vi "PID (DBL Array).vi"(6 "reinitialize? (F)":bool, 7 "output range":cluster{"output high":dbl, "output low":dbl}[](array[cluster])=[{"output high"=100.0, "output low"=-100.0}] {"output low" format="%.2f"; "output high" format="%.2f"}, 8 "dt (s)":dbl=-1.0 format="%.3f", 9 "PID gains":T1(array[cluster])=[{"proportional gain (Kc)"=1.0, "integral time (Ti, min)"=0.01, "derivative time (Td, min)"=0.0}] {"derivative time (Td, min)" format="%.3f"; "integral time (Ti, min)" format="%.3f"; "proportional gain (Kc)" format="%.3f"}, 10 "process variable":dbl[](array[numeric])=[0.0] format="%.2f", 11 "setpoint":dbl[](array[numeric])=[0.0] format="%.2f") -> (0 "dt out (s)":dbl format="%.3f", 3 "output":dbl[](array[numeric]) format="%.2f")   [LabVIEW 2020, in "NI_PID_pid.lvlib"]
doc: "Implements a PID controller using a PID algorithm for simple PID applications or high speed control applications that require an efficient algorithm. The PID algorithm features control output range limiting with integrator anti-windup and bumpless controller output for PID gain changes. Use the DBL instance of this VI to implement a single control loop. Use the DBL Array instance to implement parallel multi-loop control."
uses:
  <vilib>/addons/control/pid/NI_PID_pid.lvlib
  <vilib>/addons/control/pid/lvpidtkt.dll
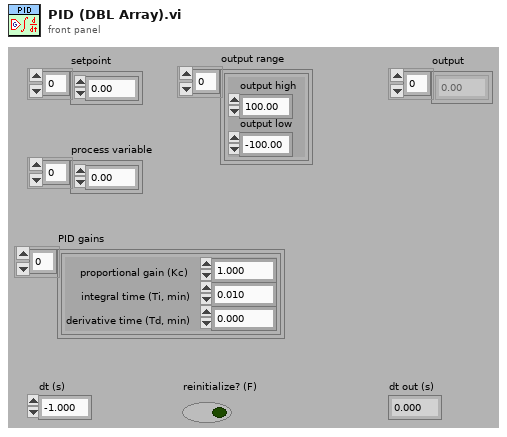
[diagram p1: front panel]
types:
  T1 = cluster{"proportional gain (Kc)":dbl, "integral time (Ti, min)":dbl, "derivative time (Td, min)":dbl}[]
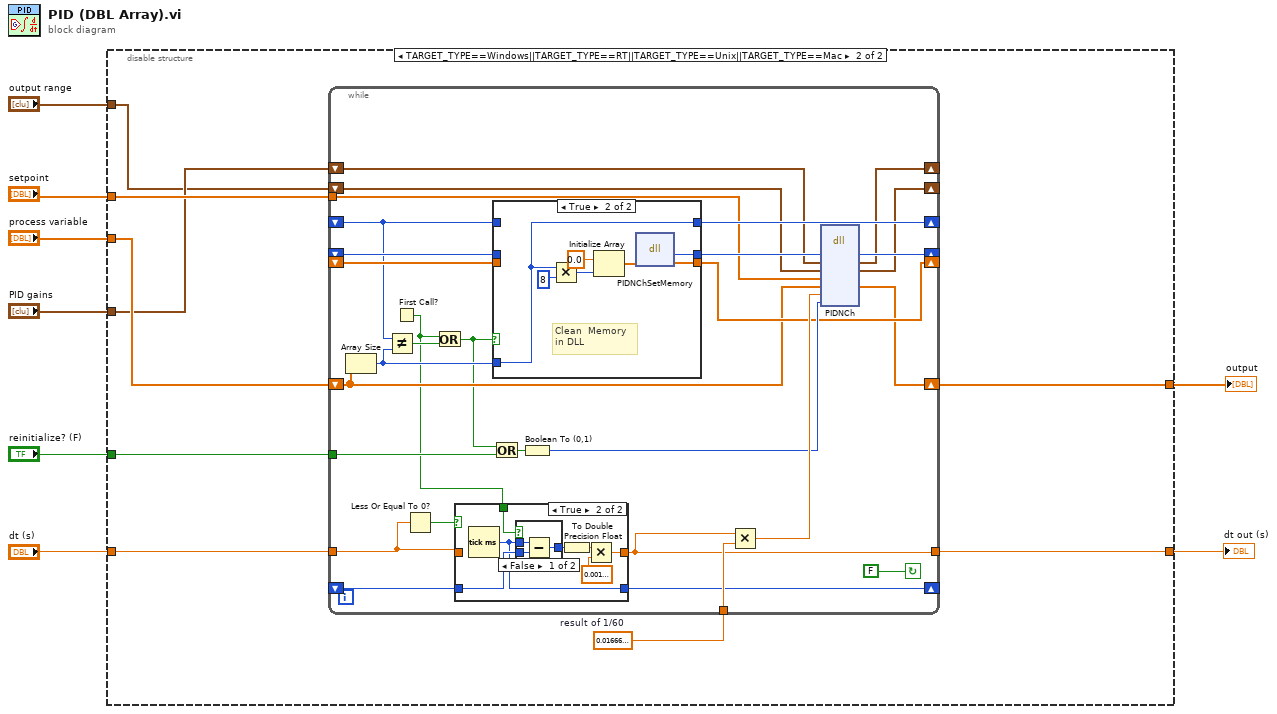
[diagram p0: block diagram]
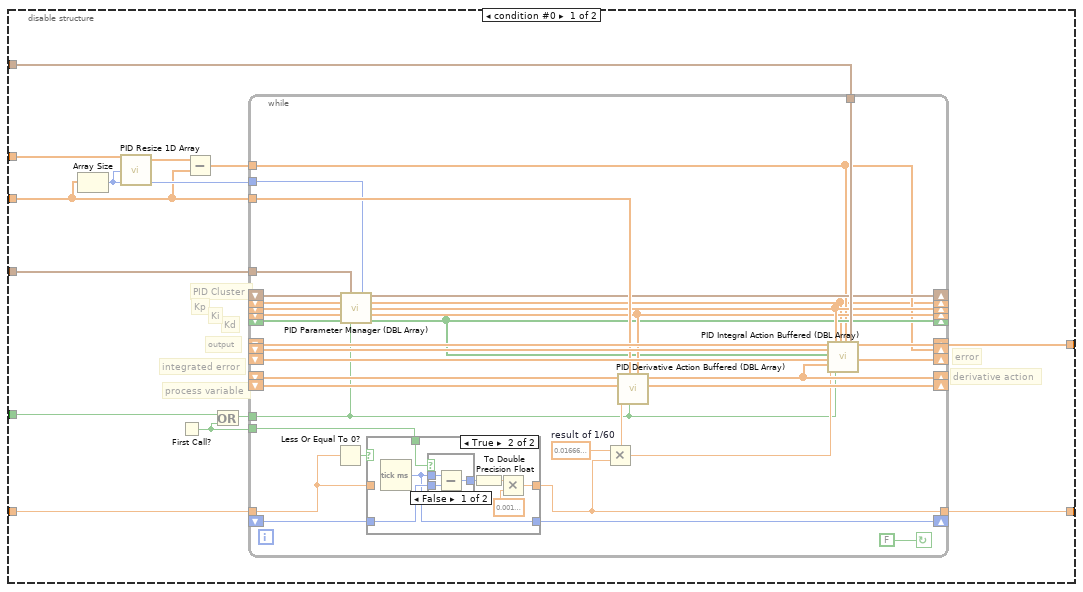
[diagram p2: hidden frame]
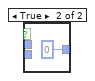
[diagram p4: hidden frame]
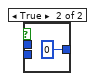
[diagram p6: hidden frame]
diagram:
  n1 = disable-structure shown="TARGET_TYPE==Windows||TARGET_TYPE==RT||TARGET_TYPE==Unix||TARGET_TYPE==Mac" {
    disable-tunnel: "reinitialize? (F)" -> [w21 w72]
    disable-tunnel: [w20 w75] -> w7
    disable-tunnel: [w19 w76] -> w6
    disable-tunnel: "dt (s)" -> [w18 w77]
    disable-tunnel: "output range" -> [w15 w69]
    disable-tunnel: "setpoint" -> [w13 w74]
    disable-tunnel: "process variable" -> [w10 w73]
    disable-tunnel: "PID gains" -> [w14 w70]
    frame condition #0 {
      # "Kd"
      # "Ki"
      # "Kp"
      # "PID Cluster"
      # "integrated error"
      # "error"
      # "output"
      # "process variable"
      # "derivative action"
      n2 = Array Size(array=w10) -> (size(s)=w12:i32)
      n3 = call <vilib>:"PID Resize 1D Array.vi"("array size"=w12, "input array"=w13) -> ("output array"=w11:dbl[])  [unwired: 3 in]
      n4 = First Call?() -> (First Call?: T/F=w16:bool)
      n5 = Subtract(x=w11, y=w10) -> (x-y=w9:dbl[])
      n6 = Or(x=w21, y=w16) -> (x .or. y?=w17:bool)
      n7 = while {
        tunnel: w17 -> [w25]
        shift-left: _ -> [w42]
        shift-right: [w41] -> _
        shift-right: [w46] -> _
        shift-left: _ -> [w47]
        shift-right: [w54] -> _
        shift-left: _ -> [w48]
        shift-right: [w53] -> w20
        shift-left: _ -> [w51]
        shift-right: [w23] -> _
        shift-left: _ -> [w52]
        shift-right: [w50] -> _
        shift-left: _ -> [w49]
        tunnel: w18 -> [w38]
        tunnel: [w40] -> w19
        tunnel: w10 -> [w36]
        tunnel: w12 -> [w24]
        tunnel: w15 -> [w43]
        tunnel: w16 -> [w37]
        shift-right: [w26] -> _
        shift-left: _ -> [w35]
        shift-right: [w27] -> _
        shift-left: _ -> [w34]
        shift-right: [w28] -> _
        shift-left: _ -> [w33]
        shift-right: [w22] -> _
        shift-left: _ -> [w32]
        shift-right: [w31] -> _
        shift-left: _ -> [w30]
        tunnel: w14 -> [w29]
        tunnel: w9 -> [w23]
        stop <- FALSE continue-if-true
        w44 = 0.016666666666666666  # result of 1/60
        n8 = Less Or Equal To 0?(x=w38) -> (x <= 0?=w39:bool)
        n9 = call <vilib>:"PID Parameter Manager (DBL Array).vi"("previous PID gains"=w30, "PID gains"=w29, "process variable size"=w24, "previous Kp"=w32, "previous Ki"=w33, "previous Kd"=w34, "previous PID Gains equal ?"=w35, "initialize"=w25) -> ("PID Parameter Out"=w31:T1, "Kp"=w22:dbl[], "Ki"=w28:dbl[], "Kd"=w27:dbl[], "PID Gains equal ?"=w26:bool[])  [unwired: 2 in, 1 out]
        n10 = case shown="True" w39 {
          tunnel: [w57 w61] -> w40
          tunnel: w42 -> [w56 w60]
          tunnel: [w56 w59] -> w41
          tunnel: w38 -> [w57 _]
          tunnel: w37 -> [_ w58]
          frame False {
          }
          frame True {
            n11 = Tick Count (ms)() -> (millisecond timer value=w59:u32)
            n12 = case shown="False" w58 {
              tunnel: [w67 u32 0] -> w63
              tunnel: w60 -> [w66 _]
              tunnel: w59 -> [w65 _]
              frame False {
                n13 = Subtract(x=w65, y=w66) -> (x-y=w67:u32)
              }
              frame True {
              }
            }
            n14 = To Double Precision Float(number=w63) -> (double precision float=w62:dbl)
            n15 = Multiply(x=w62, y=0.0010000000474974513) -> (x*y=w61:dbl)
          }
        }
        n16 = Multiply(x=w44, y=w40) -> (x*y=w45:dbl)
        n17 = call <vilib>:"PID Derivative Action Buffered (DBL Array).vi"("Kd"=w27, "initialize (F)"=w25, "process variable"=w36, "dt (min)"=w45, "previous  process variable"=w48, "previous derivative action"=w47) -> ("process variable buffer"=w54:dbl[], "derivative action"=w46:dbl[])  [unwired: 4 in]
        n18 = call <vilib>:"PID Integral Action Buffered (DBL Array).vi"("previous output"=w51, "previous error"=w52, "PID Gains equal?"=w26, "previous integrated error"=w49, "previous derivative action"=w46, "dt (min)"=w45, "Ki"=w28, "initialize (F)"=w25, "proportional action"=w22, "error"=w23, "output range"=w43) -> ("output"=w53:dbl[], "integrated error out"=w50:dbl[])  [unwired: 7 in]
      }
    }
    frame condition #1 (active) {
      w71 = 0.016666666666666666  # result of 1/60
      n19 = while {
        shift-right: [w81] -> _
        shift-left: _ -> [w82]
        shift-right: [w101] -> _
        shift-left: _ -> [w102]
        shift-right: [w99] -> _
        shift-left: _ -> [w98]
        shift-right: [w97] -> _
        shift-left: _ -> [w95]
        shift-right: [w91] -> _
        shift-left: w70 -> [w93]
        shift-right: [w90] -> _
        shift-left: w69 -> [w92]
        shift-right: [w88] -> w75
        shift-left: w73 -> [w89]
        tunnel: w77 -> [w80]
        tunnel: w74 -> [w86]
        tunnel: [w78] -> w76
        tunnel: w72 -> [w85]
        tunnel: w71 -> [w84]
        stop <- FALSE continue-if-true
        n20 = Array Size(array=w89) -> (size(s)=w96:i32)
        n21 = Not Equal?(x=w95, y=w96) -> (x != y?=w94:bool)
        n22 = First Call?() -> (First Call?: T/F=w79:bool)
        n23 = Less Or Equal To 0?(x=w80) -> (x <= 0?=w83:bool)
        n24 = Or(x=w79, y=w94) -> (x .or. y?=w87:bool)
        n25 = case shown="True" w83 {
          tunnel: [w108 w112] -> w78
          tunnel: w82 -> [w107 w111]
          tunnel: [w107 w110] -> w81
          tunnel: w80 -> [w108 _]
          tunnel: w79 -> [_ w109]
          frame False {
          }
          frame True {
            n26 = Tick Count (ms)() -> (millisecond timer value=w110:u32)
            n27 = case shown="False" w109 {
              tunnel: [w118 u32 0] -> w114
              tunnel: w111 -> [w117 _]
              tunnel: w110 -> [w116 _]
              frame False {
                n28 = Subtract(x=w116, y=w117) -> (x-y=w118:u32)
              }
              frame True {
              }
            }
            n29 = To Double Precision Float(number=w114) -> (double precision float=w113:dbl)
            n30 = Multiply(x=w113, y=0.0010000000474974513) -> (x*y=w112:dbl)
          }
        }
        n31 = Or(x=w87, y=w85) -> (x .or. y?=w104:bool)
        n32 = case shown="True" w87 {
          tunnel: [w122 w127] -> w100
          tunnel: w102 -> [w122 _]
          tunnel: [w121 w126] -> w99
          tunnel: w98 -> [w121 _]
          tunnel: w95 -> [w120 _]
          tunnel: w96 -> [_ w123]
          tunnel: [w120 w123] -> w97
          frame False {
          }
          frame True {
            # "Clean  Memory\nin DLL"
            n33 = Multiply(x=w123, y=8 ("dimension size")) -> (x*y=w124:i32)
            n34 = Initialize Array(0.0 ("element"), w124) -> (w128:dbl[])
            n35 = dll-call lib="e:/builds/penguin/labview/branches/2020/dev/dist/vi.lib/addons/control/pid/lvpidtkt.*" fn="PIDNChSetMemory"("historyData"=w128) -> ("return type"=w127:u64, "historyData"=w126:dbl[])  [unwired: 3 in, 2 out]
          }
        }
        n36 = Boolean To (0,1)(Boolean=w104) -> (0, 1=w103:i16)
        n37 = Multiply(x=w78, y=w84) -> (x*y=w105:dbl)
        n38 = dll-call lib="e:/builds/penguin/labview/branches/2020/dev/dist/vi.lib/addons/control/pid/lvpidtkt.*" fn="PIDNCh"("historyData"=w100, "PIDGains"=w93, "outputRange"=w92, "setpoints"=w86, "processVariables"=w89, "dt"=w105, "init"=w103) -> ("historyData"=w101:u64, "PIDGains"=w91:T1, "outputRange"=w90:cluster{"output high":dbl, "output low":dbl}[], "processVariables"=w88:dbl[])  [unwired: 5 in, 4 out]
      }
    }
  }
  "output" <- w7
  "dt out (s)" <- w6
